vi "Chronos TDMS Filename from Timestamp.vi"(8 "error in (no error)":errorcluster, 9 "Path to log":path, 10 "suffix":string, 11 "time stamp":timestamp) -> (0 "error out":errorcluster, 2 "day of year":i32, 3 "path":path)   [LabVIEW 2024]
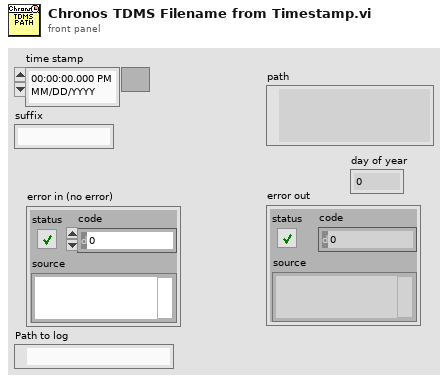
[diagram p1: front panel]
types:
  T1 = typedef "LVDateTimeRec.ctl" = cluster{"fractional second":dbl, "second":i32, "minute":i32, "hour":i32, "day of month":i32, "month":i32, "year":i32, "day of week":i32, "day of year":i32, "DST":i32}
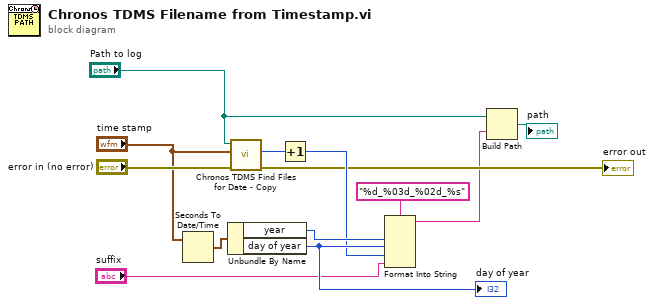
[diagram p0: block diagram]
diagram:
  n1 = Seconds To Date/Time(time stamp (now)="time stamp") -> (date time rec=w13:T1)  [unwired: 1 in]
  n2 = Unbundle By Name(w13) -> ("year"=w11:i32, "day of year"=w10:i32)
  "day of year" <- w10
  n3 = call "Chronos TDMS Find Files for Date - Copy.vi"("error in (no error)"="error in (no error)", "time stamp"="time stamp", "path"="Path to log") -> ("error out"=→"error out":errorcluster, "last file ID"=w6:i32)  [unwired: 6 in, 1 out]
  n4 = Increment(x=w6) -> (x+1=w5:i32)
  n5 = Format Into String(format string="%d_%03d_%02d_%s", w11, w10, w5, "suffix") -> (resulting string=w2:string)  [unwired: 2 in, 1 out]
  n6 = Build Path(base path="Path to log", name or relative path=w2) -> (appended path=→"path":path)
